vi "CreateProduct.vi"(8 "error in (no error)":errorcluster, 11 "CreatorA":refnum<class "CreatorA.lvclass">) -> (0 "error out":errorcluster, 2 "Product":refnum<class "Product.lvclass">, 3 "CreatorA":refnum<class "CreatorA.lvclass">)   [LabVIEW 2020, in "FactoryMethod.lvlib" / "FactoryMethodLazyEvaluation.lvlib" / "CreatorA.lvclass"]
uses:
  CreatorA.lvclass
  Product/Product.lvclass
  ProductA/ProductA.lvclass
  E:/Francesco/GitHub/Design-Patterns-GoF_-_NI-LV/Creational/FactoryMethod/GoF_Example/FactoryMethodLazyEvaluation/Product/Product.lvclass
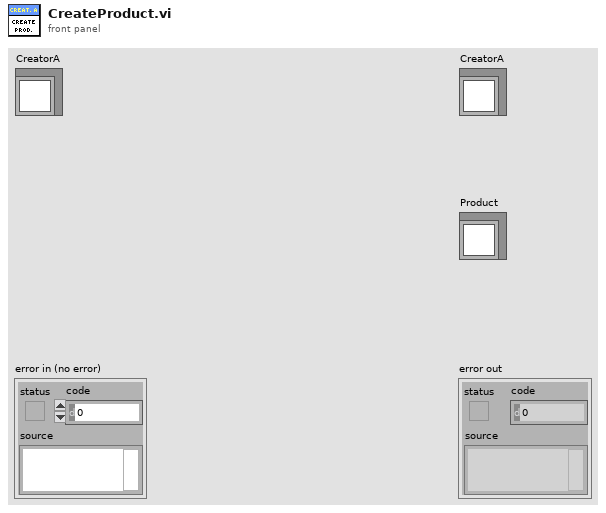
[diagram p1: front panel]
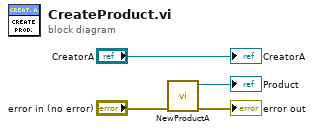
[diagram p0: block diagram]
diagram:
  n1 = call "NewProductA.vi"("error in (no error)"="error in (no error)") -> ("error out"=→"error out":errorcluster, "ProductA"=→"Product":refnum<class "ProductA.lvclass">)  [unwired: 9 in]
  "CreatorA" <- "CreatorA"
